vi "Read (Multiple Waveforms).vi"(8 "error in (no error)":errorcluster, 9 "Maximum Time (10000ms)":u32=10000, 10 "Channels":u16[](array[ring])=[0] items=["Channel 1", "Channel 2", "Channel 3", "Channel 4", "Math", "Reference 1", "Reference 2", "Reference 3", "Reference 4"], 11 "VISA resource name":refnum<visa-resource-name>) -> (0 "error out":errorcluster, 2 "Waveform Data":waveform(dbl)[](graph), 3 "VISA resource name out":refnum<visa-resource-name>)   [LabVIEW 2009, in "Tektronix DPO MSO 2000 4000 Series.lvlib"]
doc: "Initiates an acquisition on all channels that you enabled with the <B>Configure Channel</B> VI. The VI waits for the acquisition to complete and returns the waveform for the <B>Channels</B> you specified. The <B>Timeout</B> control specifies the maximum time to wait for operation complete in milliseconds. If the oscilloscope did not complete the acquisition within the time period you specify with the Timeout parameter, the VI returns a timeout error. A common cause for a timeout error is the acquisition was not triggered. For example, the trigger level is out of range of the waveform."
uses:
  <instrlib>/Tektronix DPO MSO 2000 4000 Series/Tektronix DPO MSO 2000 4000 Series.lvlib
  <instrlib>/Tektronix DPO MSO 2000 4000 Series/Public/Data/Data_Low Level/Fetch Waveform (Waveform Data Type).vi
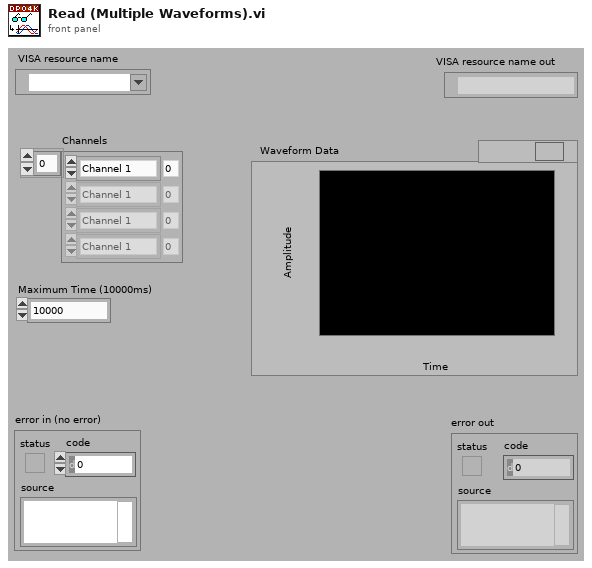
[diagram p1: front panel]
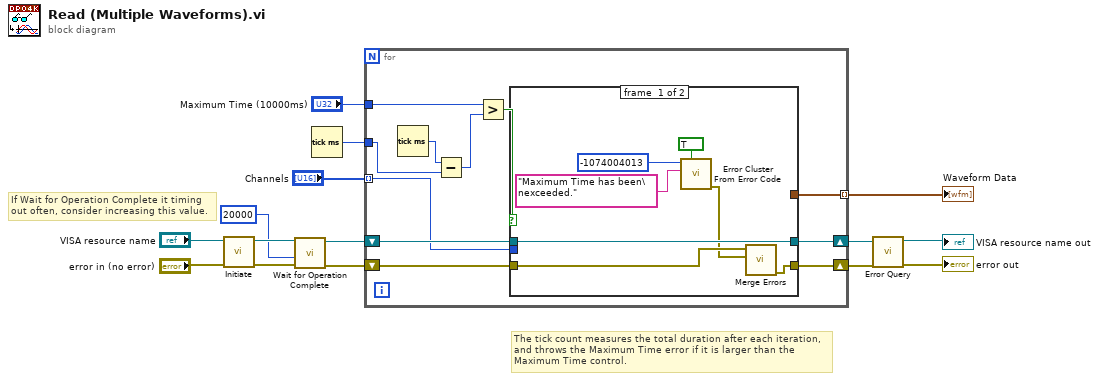
[diagram p0: block diagram]
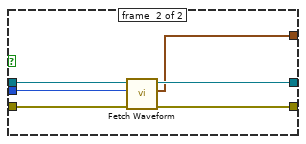
[diagram p2: hidden frame]
diagram:
  # "If Wait for Operation Complete it timing out often, consider increasing this value."
  # "The tick count measures the total duration after each iteration, and throws the Maximum Time error if it is larger than the Maximum Time control."
  n1 = call <instrlib>:"Initiate.vi"("error in (no error)"="error in (no error)", "VISA resource name"="VISA resource name") -> ("error out"=w6:errorcluster, "VISA resource name out"=w7:refnum<visa-resource-name>)  [unwired: 8 in]
  n2 = call <instrlib>:"Wait for Operation Complete.vi"("error in (no error)"=w6, "Maximum Time (10000ms)"=u32 20000, "VISA resource name"=w7) -> ("error out"=w4:errorcluster, "VISA resource name out"=w5:refnum<visa-resource-name>)  [unwired: 7 in]
  n3 = Tick Count (ms)() -> (millisecond timer value=w2:u32)
  n4 = for {
    shift-right: [w24] -> w14
    shift-left: w5 -> [w25]
    shift-right: [w23] -> w13
    shift-left: w4 -> [w26]
    tunnel: "Channels" -> [w22] mode=indexing
    tunnel: [w21] -> w10 mode=indexing
    tunnel: w2 -> [w19]
    tunnel: "Maximum Time (10000ms)" -> [w18]
    n5 = Tick Count (ms)() -> (millisecond timer value=w20:u32)
    n6 = Subtract(x=w20, y=w19) -> (x-y=w17:u32)
    n7 = Greater?(x=w18, y=w17) -> (0:w16:bool)
    n8 = case shown="True" w16 {
      tunnel: w26 -> [w28 w39]
      tunnel: w25 -> [w33 w38]
      tunnel: [w33 w37] -> w24
      tunnel: [w29 w36] -> w23
      tunnel: w22 -> [_ w35]
      tunnel: [_ w34] -> w21
      frame #0 {
        n9 = call <vilib>:"Error Cluster From Error Code.vi"("show call chain? (False)"=TRUE, "error message (\"\")"="Maximum Time has been\nexceeded." ("error message (\"\")"), "error code (0)"=-1074004013) -> ("error out"=w27:errorcluster)  [unwired: 6 in]
        n10 = call <vilib>:"Merge Errors.vi"("error in 2 (no error)"=w27, "error in 1 (no error)"=w28) -> ("error out"=w29:errorcluster)  [unwired: 5 in]
      }
      frame #1 {
        n11 = call-poly <instrlib>:"Fetch Waveform.vi"("error in (no error)"=w39, "Channel (0: Channel 1)"=w35, "VISA resource name"=w38) -> ("error out"=w36:errorcluster, "Waveform Data"=w34:waveform(dbl), "VISA resource name out"=w37:refnum<visa-resource-name>)  [unwired: 6 in]
      }
    }
  }
  "Waveform Data" <- w10
  n12 = call <instrlib>:"Error Query.vi"("error in (no error)"=w13, "VISA resource name"=w14) -> ("error out"=→"error out":errorcluster, "VISA resource name out"=→"VISA resource name out":refnum<visa-resource-name>)  [unwired: 6 in, 2 out]
